vi "Begin.vi"(8 "error in":errorcluster) -> (0 "error out":errorcluster)   [LabVIEW 2014]
doc: "Called before other user functions, this VI is expected to open initial I/O refnums, load in file data, and do all program initialization. Notice that the <B>error out</B> terminal is simply used for data flow. Wiring it to other structures or subVIs ensures that this VI runs first."
uses:
  <vilib>/Rock Robotics/WPI/DriverStation/WPI_DriverStationRobotMode2.ctl
  <vilib>/Rock Robotics/WPI/Joystick/WPI_JoystickDeviceEnum.ctl
  <vilib>/Rock Robotics/WPI/SafetyOutput/WPI_SafetyOutputConfigMenu.ctl
  <vilib>/Rock Robotics/SystemInterfaces/AI/FPGA_AIGyroChannel.ctl
  <vilib>/Rock Robotics/SystemInterfaces/DIO/FPGA_DIOChannel.ctl
  <vilib>/Rock Robotics/WPI/Encoder/WPI_EncoderType.ctl
  <vilib>/Rock Robotics/WPI/Solenoid/WPI_SolenoidChannel.ctl
  <vilib>/Rock Robotics/WPI/CAN/TalonSRX/WPI_CANTalonSRX_APIControlMode.ctl
  <vilib>/Rock Robotics/SystemInterfaces/AI/FPGA_AIChannel.ctl
  Robot Global Data.vi
  <vilib>/Rock Robotics/Network Tables/SD Write String Array.vi
  <vilib>/Rock Robotics/WPI/MotorControl/WPI_MotorControlOpenCANTalonSRX.vi
  <vilib>/Rock Robotics/WPI/Counter/WPI_CounterDigitalInputToDigitalSource.vi
  <vilib>/Rock Robotics/WPI/Solenoid/WPI_SolenoidOpenSingle.vi
  <vilib>/Rock Robotics/WPI/Compressor/WPI_CompressorGetSetRefNum.vi
  <vilib>/Rock Robotics/WPI/RobotDrive/WPI_RobotDriveOpen2MotorWithCANTalonSRX.vi
  <vilib>/Rock Robotics/WPI/Switch/WPI_SwitchOpenLimit.vi
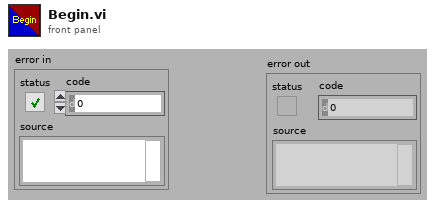
[diagram p1: front panel]
types:
  T1 = typedef "WPI_SolenoidChannel.ctl" = enum8{"Solenoid 0", "Solenoid 1", "Solenoid 2", "Solenoid 3", "Solenoid 4", "Solenoid 5", "Solenoid 6", "Solenoid 7", "Invalid"}
  T2 = typedef "FPGA_DIOChannel.ctl" = enum8{"DIO 0", "DIO 1", "DIO 2", "DIO 3", "DIO 4", "DIO 5", "DIO 6", "DIO 7", "DIO 8", "DIO 9", "DIO MXP 0", "DIO MXP 1", "DIO MXP 2", "DIO MXP 3", "DIO MXP 4", "DIO MXP 5", "DIO MXP 6", "DIO MXP 7", "DIO MXP 8", "DIO MXP 9", "DIO MXP 10", "DIO MXP 11", "DIO MXP 12", "DIO MXP 13", "DIO MXP 14", "DIO MXP 15", "Invalid"}
  T3 = typedef "FPGA_AIChannel.ctl" = enum8{"AI 0", "AI 1", "AI 2", "AI 3", "AI MXP 0", "AI MXP 1", "AI MXP 2", "AI MXP 3", "Invalid"}
  T4 = typedef "WPI_CANTalonSRX_APIControlMode.ctl" = enum8{"Percent VBus", "Speed", "Position", "Slave", "Unchanged / Invalid"}
  T5 = typedef "WPI_EncoderType.ctl" = enum16{"1x", "2x", "4x"}
  T6 = typedef "FPGA_AIGyroChannel.ctl" = enum8{"AI 0", "AI 1", "Invalid"}
  T7 = typedef "WPI_JoystickDeviceEnum.ctl" = enum16{"USB 0", "USB 1", "USB 2", "USB 3", "USB 4", "USB 5"}
  T8 = typedef "WPI_SafetyOutputConfigMenu.ctl" = enum16{"Enable", "Disable"}
  T9 = typedef "WPI_DriverStationRobotMode2.ctl" = enum16{"Autonomous Disabled", "Autonomous Enabled", "Teleop Disabled", "Teleop Enabled", "Disconnected", "Finish", "Test Disabled", "Test Enabled", "Emergency Stopped"}
  T10 = typedef "WPI_PotentiometerDevRef.ctl" = cluster{"DevStatus":errorcluster, "Controller":T11, "Analog Channel":T3, "Invert Output":bool}
  T11 = typedef "FPGA_TypedefAnalogModule.ctl" = enum16{"Controller 1"}
  T12 = typedef "WPI_JoystickDevRef.ctl" = cluster{"Device":T7}
  T13 = typedef "WPI_DigitalInputDevRef.ctl" = cluster{"DevStatus":errorcluster, "DIO Channel":T2, "Controller":T14}
  T14 = typedef "FPGA_TypedefDigitalModule.ctl" = enum16{"Controller 1"}
  T15 = typedef "WPI_SwitchDevRef.ctl" = cluster{"DevStatus":errorcluster, "DIO Channel":T2, "Controller":T14, "CntIndex":T16, "Normally Closed":bool}
  T16 = typedef "FPGA_CounterCtrSystemIndex.ctl" = enum8{"Ctr 0", "Ctr 1", "Ctr 2", "Ctr 3", "Ctr 4", "Ctr 5", "Ctr 6", "Ctr 7", "Invalid"}
  T17 = typedef "FPGA_CounterEncoderSourceConvertionLVSourceType.ctl" = cluster{"DevStatus":errorcluster, "AnalogTriggerMode?":bool, "DigitalMode":cluster{"Controller":T14, "DIO Channel":T18}, "AnalogTriggerMode":cluster{"AnalogTriggerIndex":T19, "OutputType":T20}}
  T18 = typedef "FPGA_DIODigitalSourceChannel.ctl" = enum8{"DIO 0", "DIO 1", "DIO 2", "DIO 3", "DIO 4", "DIO 5", "DIO 6", "DIO 7", "DIO 8", "DIO 9", "DIO MXP 0", "DIO MXP 1", "DIO MXP 2", "DIO MXP 3", "DIO MXP 4", "DIO MXP 5", "DIO MXP 6", "DIO MXP 7", "DIO MXP 8", "DIO MXP 9", "DIO MXP 10", "DIO MXP 11", "DIO MXP 12", "DIO MXP 13", "DIO MXP 14", "DIO MXP 15", "Disabled"}
  T19 = typedef "FPGA_AnalogTriggerIndex.ctl" = enum8{"Trig 0", "Trig 1", "Trig 2", "Trig 3", "Trig 4", "Trig 5", "Trig 6", "Trig 7", "Invalid"}
  T20 = typedef "FPGA_AnalogTriggerOutType.ctl" = enum16{"InWindow", "TriggerState", "Rising", "Falling"}
  T21 = typedef "WPI_SolenoidDevRef.ctl" = cluster{"DevStatus":errorcluster, "Pneumatics Control Module":u8, "Forward Solenoid Channel":T1, "Reverse Solenoid Channel":T1}
  T22 = typedef "WPI_GyroDevRef.ctl" = cluster{"DevStatus":errorcluster, "Analog Module":T11, "Analog Channel":T3, "Offset":dbl, "Gain (VoltsPerDegree/Second)":dbl}
  T23 = typedef "WPI_MotorControlDeviceRef.ctl" = cluster{"DeviceStatus":errorcluster, "Type":T24, "PWM":cluster{"Controller":T14, "PWM Channel":T25, "DeadBand":T26}, "CAN":cluster{"Device Number":u8, "Control Mode":T27, "Semaphore":T28, "Max Vout":dbl, "TalonSRX Control Mode":T4}, "Invert":bool, "TransformRef":T29, "InvTransformRef":T29}
  T24 = typedef "WPI_MotorControlType.ctl" = enum16{"PWM", "CAN", "CANTalonSRX"}
  T25 = typedef "FPGA_DIOPWMChannel.ctl" = enum8{"PWM 0", "PWM 1", "PWM 2", "PWM 3", "PWM 4", "PWM 5", "PWM 6", "PWM 7", "PWM 8", "PWM 9", "PWM MXP 0", "PWM MXP 1", "PWM MXP 2", "PWM MXP 3", "PWM MXP 4", "PWM MXP 5", "PWM MXP 6", "PWM MXP 7", "PWM MXP 8", "PWM MXP 9", "Invalid"}
  T26 = typedef "WPI_PWMDeadband.ctl" = cluster{"Name":string, "maxPositivePwm":i32, "minPositivePwm":i32, "centerPwm":i32, "maxNegativePwm":i32, "minNegativePwm":i32, "angularRange":u16}
  T27 = typedef "WPI_CANJaguar_ControlMode.ctl" = enum8{"Percent VBus", "Current", "Speed", "Position", "Voltage"}
  T28 = typedef "Semaphore RefNum" = refnum<k1>
  T29 = typedef "WPI_PWMTransform_ConPane.ctl" = refnum<vi>
  T30 = typedef "WPI_EncoderDevRef.ctl" = cluster{"DevStatus":errorcluster, "EncoderIndex":T31, "CounterIndex":T16, "DistancePerCount":dbl, "Decoding Type":T5}
  T31 = typedef "FPGA_EncoderIdx.ctl" = enum8{"Enc 0", "Enc 1", "Enc 2", "Enc 3", "Enc 4", "Enc 5", "Enc 6", "Enc 7", "Invalid"}
  T32 = typedef "WPI_RobotDriveDevRef.ctl" = cluster{"DevStatus":errorcluster, "Motors[]":T23[], "Square Inputs":bool, "Max Output":dbl}
  T33 = typedef "WPI_CompressorDevRef.ctl" = cluster{"DevStatus":errorcluster, "Pneumatics Control Module":u8}
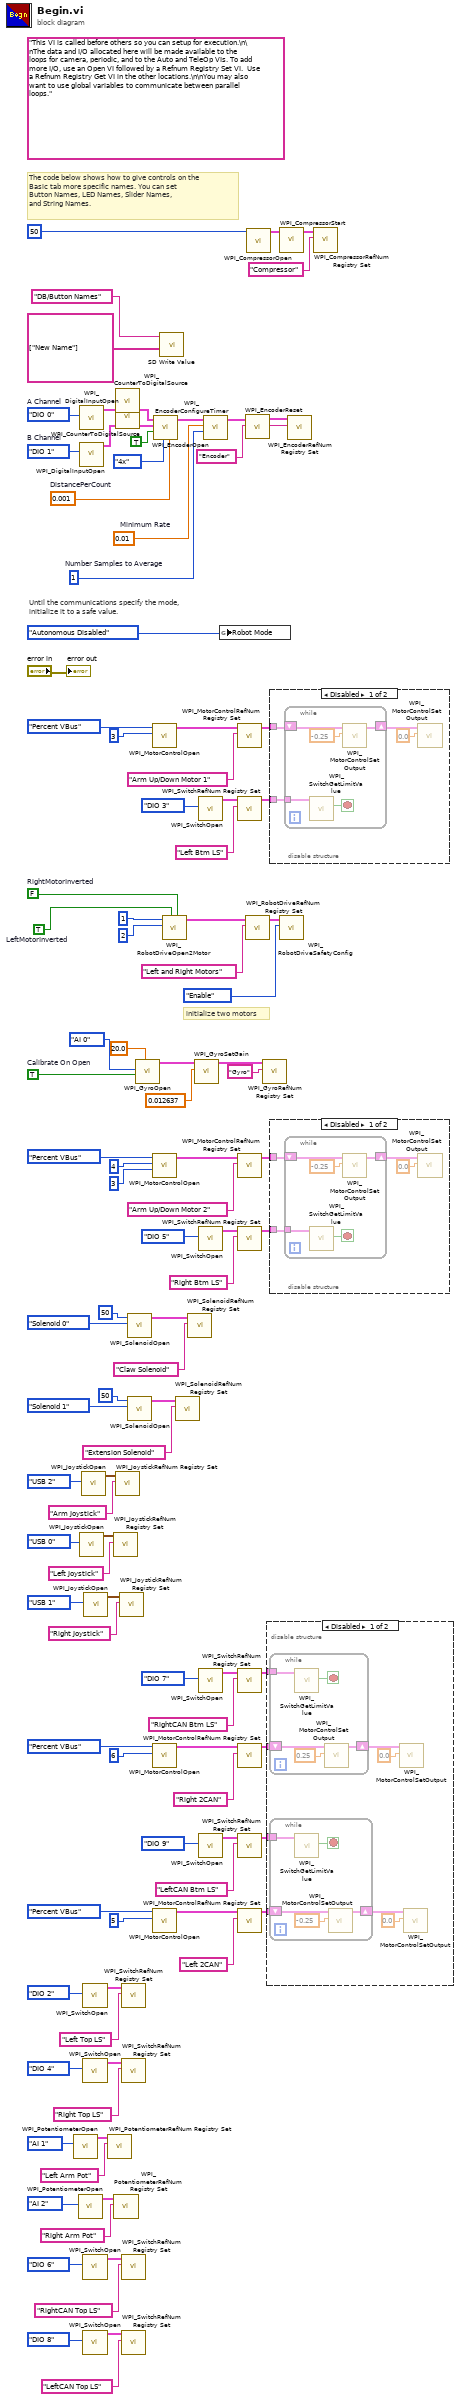
[diagram p0: block diagram]
diagram:
  w74 = u8 1  # Number Samples to Average
  w75 = 0.01  # Minimum Rate
  w77 = 0.001  # DistancePerCount
  w85 = FPGA_DIOChannel."DIO 1"  # B Channel
  w84 = FPGA_DIOChannel."DIO 0"  # A Channel
  w87 = TRUE  # Calibrate On Open
  w97 = TRUE  # LeftMotorInverted
  w64 = FALSE  # RightMotorInverted
  (unwired) "This VI is called before others so you can setup for execution.\n\nThe data and I/O allocated here will be made available to the loops for camera, periodic, and to the Auto and TeleOp VIs. To add more I/O, use an Open VI followed by a Refnum Registry Set VI.  Use a Refnum Registry Get VI in the other locations.\n\nYou may also want to use global variables to communicate between parallel loops."
  # "initialize two motors"
  # "The code below shows how to give controls on the\nBasic tab more specific names. You can set\nButton Names, LED Names, Slider Names,\nand String Names."
  # "Until the communications specify the mode,\ninitialize it to a safe value."
  n1 = call <vilib>:"WPI_PotentiometerOpen.vi"("Analog Channel"=FPGA_AIChannel."AI 1") -> ("PotDevRef"=w31:T10)  [unwired: 9 in, 1 out]
  n2 = call <vilib>:"WPI_PotentiometerOpen.vi"("Analog Channel"=FPGA_AIChannel."AI 2") -> ("PotDevRef"=w28:T10)  [unwired: 9 in, 1 out]
  n3 = call <vilib>:"WPI_JoystickOpen.vi"("JoystickDevice"=WPI_JoystickDeviceEnum."USB 0") -> ("JoystickDevRef"=w108:T12)  [unwired: 10 in]
  n4 = call <vilib>:"WPI_DigitalInputOpen.vi"("DIO Channel"=w84) -> ("DigitalInputDevRef"=w81:T13)  [unwired: 2 in, 8 out]
  n5 = call <vilib>:"WPI_DigitalInputOpen.vi"("DIO Channel"=w85) -> ("DigitalInputDevRef"=w82:T13)  [unwired: 2 in, 8 out]
  n6 = call <vilib>:"WPI_JoystickOpen.vi"("JoystickDevice"=WPI_JoystickDeviceEnum."USB 2") -> ("JoystickDevRef"=w94:T12)  [unwired: 10 in]
  n7 = call-poly <vilib>:"WPI_SwitchOpen.vi"("DIO Channel"=FPGA_DIOChannel."DIO 2") -> ("SwitchDevRef"=w34:T15)  [unwired: 9 in, 1 out]
  n8 = call-poly <vilib>:"WPI_SwitchOpen.vi"("DIO Channel"=FPGA_DIOChannel."DIO 4") -> ("SwitchDevRef"=w40:T15)  [unwired: 9 in, 1 out]
  n9 = call-poly <vilib>:"WPI_SwitchOpen.vi"("DIO Channel"=FPGA_DIOChannel."DIO 6") -> ("SwitchDevRef"=w22:T15)  [unwired: 9 in, 1 out]
  n10 = call-poly <vilib>:"WPI_SwitchOpen.vi"("DIO Channel"=FPGA_DIOChannel."DIO 8") -> ("SwitchDevRef"=w16:T15)  [unwired: 9 in, 1 out]
  n11 = call <vilib>:"WPI_JoystickOpen.vi"("JoystickDevice"=WPI_JoystickDeviceEnum."USB 1") -> ("JoystickDevRef"=w102:T12)  [unwired: 10 in]
  n12 = call <vilib>:"WPI_PotentiometerRefNum Registry Set.vi"("refnum name"="Left Arm Pot", "PotDevRef"=w31) -> ()  [unwired: 8 in, 2 out]
  n13 = call <vilib>:"WPI_JoystickRefNum Registry Set.vi"("refnum name"="Left Joystick", "JoystickDevRef"=w108) -> ()  [unwired: 8 in, 2 out]
  n14 = call <vilib>:"WPI_PotentiometerRefNum Registry Set.vi"("refnum name"="Right Arm Pot", "PotDevRef"=w28) -> ()  [unwired: 8 in, 2 out]
  n15 = call-poly <vilib>:"WPI_CounterToDigitalSource.vi"("DigitalInputDevRef"=w81) -> ("Digital Source"=w80:T17)  [unwired: 6 out]
  n16 = call-poly <vilib>:"WPI_CounterToDigitalSource.vi"("DigitalInputDevRef"=w82) -> ("Digital Source"=w83:T17)  [unwired: 6 out]
  n17 = call <vilib>:"WPI_JoystickRefNum Registry Set.vi"("refnum name"="Arm Joystick", "JoystickDevRef"=w94) -> ()  [unwired: 8 in, 2 out]
  n18 = call <vilib>:"WPI_JoystickRefNum Registry Set.vi"("refnum name"="Right Joystick", "JoystickDevRef"=w102) -> ()  [unwired: 8 in, 2 out]
  n19 = call <vilib>:"WPI_SwitchRefNum Registry Set.vi"("refnum name"="Left Top LS", "SwitchDevRef"=w34) -> ()  [unwired: 8 in, 2 out]
  n20 = call <vilib>:"WPI_SwitchRefNum Registry Set.vi"("refnum name"="Right Top LS", "SwitchDevRef"=w40) -> ()  [unwired: 8 in, 2 out]
  n21 = call <vilib>:"WPI_SwitchRefNum Registry Set.vi"("refnum name"="RightCAN Top LS", "SwitchDevRef"=w22) -> ()  [unwired: 8 in, 2 out]
  n22 = call <vilib>:"WPI_SwitchRefNum Registry Set.vi"("refnum name"="LeftCAN Top LS", "SwitchDevRef"=w16) -> ()  [unwired: 8 in, 2 out]
  n23 = call-poly <vilib>:"WPI_SolenoidOpen.vi"("Solenoid Channel"=WPI_SolenoidChannel."Solenoid 0", "Pneumatics Control Module (0)"=u8 50) -> ("SolenoidDevRef"=w71:T21)  [unwired: 8 in, 1 out]
  n24 = call-poly <vilib>:"WPI_SolenoidOpen.vi"("Solenoid Channel"=WPI_SolenoidChannel."Solenoid 1", "Pneumatics Control Module (0)"=u8 50) -> ("SolenoidDevRef"=w8:T21)  [unwired: 8 in, 1 out]
  n25 = call <vilib>:"WPI_GyroOpen.vi"("Calibration Time (s)"=20.0, "Calibrate On Open"=w87, "Analog Channel"=FPGA_AIGyroChannel."AI 0") -> ("GyroDevRef"=w47:T22)  [unwired: 6 in, 2 out]
  n26 = call-poly <vilib>:"WPI_MotorControlOpen.vi"("Device Number"=u8 3, "Control Mode"=WPI_CANTalonSRX_APIControlMode."Percent VBus") -> ("MotorControlDeviceRef"=w90:T23)  [unwired: 8 in, 1 out]
  n27 = call-poly <vilib>:"WPI_MotorControlOpen.vi"("Master Device Number"=u8 3, "Device Number"=u8 4, "Control Mode"=WPI_CANTalonSRX_APIControlMode."Percent VBus") -> ("MotorControlDeviceRef"=w60:T23)  [unwired: 7 in, 1 out]
  n28 = call-poly <vilib>:"WPI_MotorControlOpen.vi"("Device Number"=u8 6, "Control Mode"=WPI_CANTalonSRX_APIControlMode."Percent VBus") -> ("MotorControlDeviceRef"=w50:T23)  [unwired: 8 in, 1 out]
  n29 = call-poly <vilib>:"WPI_MotorControlOpen.vi"("Device Number"=u8 5, "Control Mode"=WPI_CANTalonSRX_APIControlMode."Percent VBus") -> ("MotorControlDeviceRef"=w55:T23)  [unwired: 8 in, 1 out]
  n30 = call <vilib>:"WPI_EncoderOpen.vi"("DistancePerCount"=w77, "Decoding Type"=WPI_EncoderType."4x", "Invert Direction (False)"=TRUE, "BSource"=w83, "ASource"=w80) -> ("EncoderDevRef"=w76:T30)  [unwired: 3 in, 3 out]
  n31 = call-poly <vilib>:"SD Write Value.vi"("String Array"=string[] ["New Name"], "Name"="DB/Button Names") -> ()  [unwired: 8 in, 2 out]
  n32 = call-poly <vilib>:"WPI_RobotDriveOpen2Motor.vi"("Right Motor Inverted"=w64, "Left Motor Inverted"=w97, "Right Motor"=u8 2, "Left Motor"=u8 1) -> ("RobotDriveDevRef"=w99:T32)  [unwired: 6 in, 1 out]
  n33 = call <vilib>:"WPI_SolenoidRefNum Registry Set.vi"("refnum name"="Extension Solenoid", "SolenoidDevRef"=w8) -> ()  [unwired: 8 in, 2 out]
  n34 = call <vilib>:"WPI_SolenoidRefNum Registry Set.vi"("refnum name"="Claw Solenoid", "SolenoidDevRef"=w71) -> ()  [unwired: 8 in, 2 out]
  n35 = call <vilib>:"WPI_GyroSetGain.vi"("Gain (VoltsPerDegree/Second)"=0.012637, "GyroDevRef"=w47) -> ("GyroDevRef"=w45:T22)  [unwired: 8 in, 1 out]
  n36 = call-poly <vilib>:"WPI_SwitchOpen.vi"("DIO Channel"=FPGA_DIOChannel."DIO 3") -> ("SwitchDevRef"=w37:T15)  [unwired: 9 in, 1 out]
  n37 = call-poly <vilib>:"WPI_SwitchOpen.vi"("DIO Channel"=FPGA_DIOChannel."DIO 5") -> ("SwitchDevRef"=w43:T15)  [unwired: 9 in, 1 out]
  n38 = call-poly <vilib>:"WPI_SwitchOpen.vi"("DIO Channel"=FPGA_DIOChannel."DIO 7") -> ("SwitchDevRef"=w25:T15)  [unwired: 9 in, 1 out]
  n39 = call-poly <vilib>:"WPI_SwitchOpen.vi"("DIO Channel"=FPGA_DIOChannel."DIO 9") -> ("SwitchDevRef"=w19:T15)  [unwired: 9 in, 1 out]
  n40 = call <vilib>:"WPI_EncoderConfigureTimer.vi"("Number Samples to Average"=w74, "Minimum Rate"=w75, "EncoderDevRef"=w76) -> ("EncoderDevRef"=w2:T30)  [unwired: 7 in, 1 out]
  n41 = global write "Robot Global Data.vi" "Robot Mode"(WPI_DriverStationRobotMode2."Autonomous Disabled" ("Robot Mode")) -> ()
  n42 = call <vilib>:"WPI_MotorControlRefNum Registry Set.vi"("refnum name"="Arm Up/Down Motor 1", "MotorControlDevRef"=w90) -> ("MotorControlDevRef"=w14:T23)  [unwired: 8 in, 1 out]
  n43 = call <vilib>:"WPI_SwitchRefNum Registry Set.vi"("refnum name"="Left Btm LS", "SwitchDevRef"=w37) -> ("SwitchDevRef"=w13:T15)  [unwired: 8 in, 1 out]
  n44 = call <vilib>:"WPI_MotorControlRefNum Registry Set.vi"("refnum name"="Arm Up/Down Motor 2", "MotorControlDevRef"=w60) -> ("MotorControlDevRef"=w11:T23)  [unwired: 8 in, 1 out]
  n45 = call <vilib>:"WPI_SwitchRefNum Registry Set.vi"("refnum name"="Right Btm LS", "SwitchDevRef"=w43) -> ("SwitchDevRef"=w12:T15)  [unwired: 8 in, 1 out]
  n46 = call <vilib>:"WPI_SwitchRefNum Registry Set.vi"("refnum name"="RightCAN Btm LS", "SwitchDevRef"=w25) -> ("SwitchDevRef"=w5:T15)  [unwired: 8 in, 1 out]
  n47 = call <vilib>:"WPI_MotorControlRefNum Registry Set.vi"("refnum name"="Right 2CAN", "MotorControlDevRef"=w50) -> ("MotorControlDevRef"=w6:T23)  [unwired: 8 in, 1 out]
  n48 = call <vilib>:"WPI_SwitchRefNum Registry Set.vi"("refnum name"="LeftCAN Btm LS", "SwitchDevRef"=w19) -> ("SwitchDevRef"=w4:T15)  [unwired: 8 in, 1 out]
  n49 = call <vilib>:"WPI_MotorControlRefNum Registry Set.vi"("refnum name"="Left 2CAN", "MotorControlDevRef"=w55) -> ("MotorControlDevRef"=w3:T23)  [unwired: 8 in, 1 out]
  n50 = call <vilib>:"WPI_EncoderReset.vi"("EncoderDevRef"=w2) -> ("EncoderDevRef"=w1:T30)  [unwired: 9 in, 1 out]
  n51 = call <vilib>:"WPI_RobotDriveRefNum Registry Set.vi"("refnum name"="Left and Right Motors", "RobotDriveDevRef"=w99) -> ("RobotDriveDevRef"=w96:T32)  [unwired: 1 in, 8 out]
  n52 = call <vilib>:"WPI_CompressorOpen.vi"("Pneumatics Control Module (0)"=u8 50) -> ("CompressorDevRef"=w68:T33)  [unwired: 13 in, 1 out]
  n53 = call <vilib>:"WPI_GyroRefNum Registry Set.vi"("refnum name"="Gyro", "GyroDevRef"=w45) -> ()  [unwired: 8 in, 2 out]
  n54 = disable-structure shown="Disabled" {
    disable-tunnel: w6 -> [w114 _]
    disable-tunnel: w5 -> [w113 _]
    disable-tunnel: w4 -> [w112 _]
    disable-tunnel: w3 -> [w111 _]
    frame Disabled {
      n55 = while {
        shift-right: [w125] -> w118
        shift-left: w114 -> [w127]
        tunnel: w113 -> [w126]
        stop <- w128 stop-if-true
        n56 = call <vilib>:"WPI_SwitchGetLimitValue.vi"("SwitchDevRef"=w126) -> ("Switch Pressed"=w128:bool)  [unwired: 8 in, 2 out]
        n57 = call <vilib>:"WPI_MotorControlSetOutput.vi"("Output"=0.25, "MotorControlDevRef"=w127) -> ("MotorControlDevRef"=w125:T23)  [unwired: 7 in, 2 out]
      }
      n58 = while {
        shift-right: [w120] -> w115
        shift-left: w111 -> [w122]
        tunnel: w112 -> [w121]
        stop <- w123 stop-if-true
        n59 = call <vilib>:"WPI_SwitchGetLimitValue.vi"("SwitchDevRef"=w121) -> ("Switch Pressed"=w123:bool)  [unwired: 8 in, 2 out]
        n60 = call <vilib>:"WPI_MotorControlSetOutput.vi"("Output"=-0.25, "MotorControlDevRef"=w122) -> ("MotorControlDevRef"=w120:T23)  [unwired: 7 in, 2 out]
      }
      n61 = call <vilib>:"WPI_MotorControlSetOutput.vi"("Output"=0.0, "MotorControlDevRef"=w118) -> ()  [unwired: 7 in, 3 out]
      n62 = call <vilib>:"WPI_MotorControlSetOutput.vi"("Output"=0.0, "MotorControlDevRef"=w115) -> ()  [unwired: 7 in, 3 out]
    }
    frame Enabled {
    }
  }
  n63 = disable-structure shown="Disabled" {
    disable-tunnel: w14 -> [w132 _]
    disable-tunnel: w13 -> [w131 _]
    frame Disabled {
      n64 = while {
        shift-right: [w134] -> w129
        shift-left: w132 -> [w136]
        tunnel: w131 -> [w135]
        stop <- w137 stop-if-true
        n65 = call <vilib>:"WPI_SwitchGetLimitValue.vi"("SwitchDevRef"=w135) -> ("Switch Pressed"=w137:bool)  [unwired: 8 in, 2 out]
        n66 = call <vilib>:"WPI_MotorControlSetOutput.vi"("Output"=-0.25, "MotorControlDevRef"=w136) -> ("MotorControlDevRef"=w134:T23)  [unwired: 7 in, 2 out]
      }
      n67 = call <vilib>:"WPI_MotorControlSetOutput.vi"("Output"=0.0, "MotorControlDevRef"=w129) -> ()  [unwired: 7 in, 3 out]
    }
    frame Enabled {
    }
  }
  n68 = disable-structure shown="Disabled" {
    disable-tunnel: w12 -> [w141 _]
    disable-tunnel: w11 -> [w140 _]
    frame Disabled {
      n69 = while {
        shift-right: [w143] -> w138
        shift-left: w140 -> [w145]
        tunnel: w141 -> [w144]
        stop <- w146 stop-if-true
        n70 = call <vilib>:"WPI_SwitchGetLimitValue.vi"("SwitchDevRef"=w144) -> ("Switch Pressed"=w146:bool)  [unwired: 8 in, 2 out]
        n71 = call <vilib>:"WPI_MotorControlSetOutput.vi"("Output"=-0.25, "MotorControlDevRef"=w145) -> ("MotorControlDevRef"=w143:T23)  [unwired: 7 in, 2 out]
      }
      n72 = call <vilib>:"WPI_MotorControlSetOutput.vi"("Output"=0.0, "MotorControlDevRef"=w138) -> ()  [unwired: 7 in, 3 out]
    }
    frame Enabled {
    }
  }
  n73 = call <vilib>:"WPI_CompressorStart.vi"("CompressorDevRef"=w68) -> ("CompressorDevRef"=w67:T33)  [unwired: 9 in, 1 out]
  n74 = call <vilib>:"WPI_RobotDriveSafetyConfig.vi"("mode"=WPI_SafetyOutputConfigMenu."Enable", "RobotDriveDevRef"=w96) -> ()  [unwired: 8 in, 2 out]
  n75 = call <vilib>:"WPI_EncoderRefNum Registry Set.vi"("refnum name"="Encoder", "EncoderDevRef"=w1) -> ()  [unwired: 8 in, 2 out]
  n76 = call <vilib>:"WPI_CompressorRefNum Registry Set.vi"("refnum name"="Compressor", "CompressorDevRef"=w67) -> ()  [unwired: 8 in, 2 out]
  "error out" <- "error in"
